vi "IQ_ramp_test.vi"() -> ()   [LabVIEW 2013]
panel:
  in  "Q ramp length":i32
  in  "I ramp length":i32
  out "signal":i16[](graph)
  out "IQ counters":dbl[][](graph)
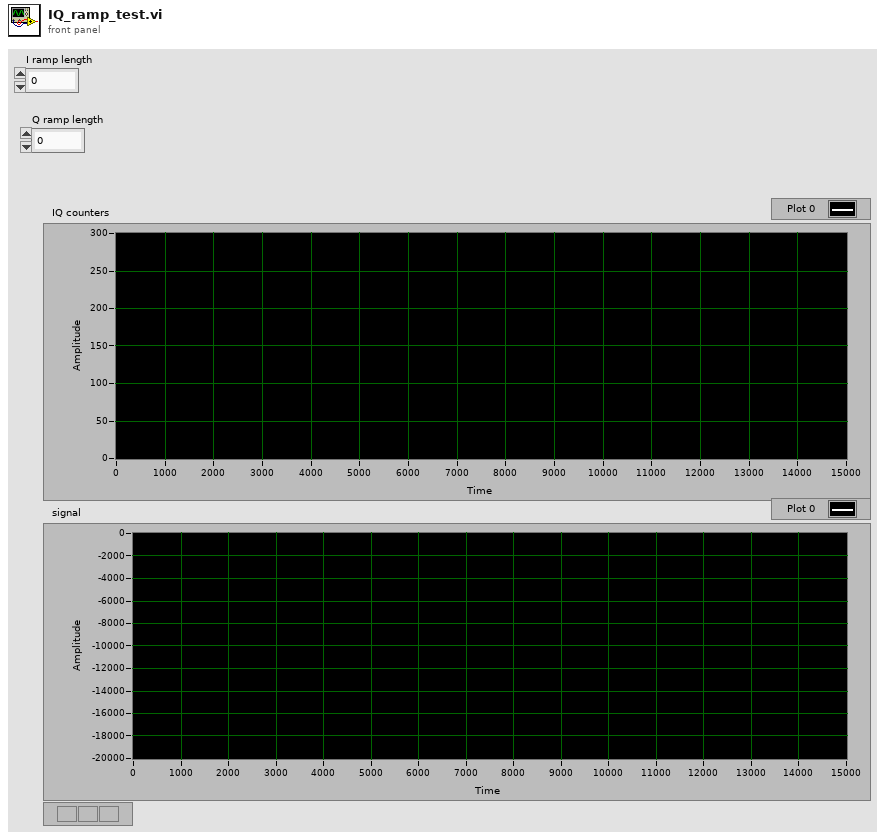
[diagram p1: front panel]
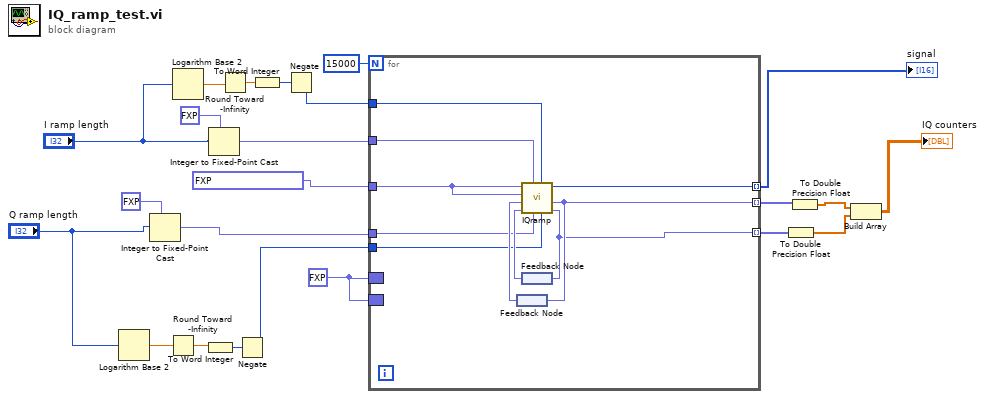
[diagram p0: block diagram]
diagram:
  w22 = fxp<+/-,32,32> 0.0 ("Q counter out")
  n1 = Logarithm Base 2(1:"Q ramp length") -> (0:w14:dbl)
  n2 = Integer to Fixed-Point Cast(fixed-point type=fxp<+/-,32,32> 0.0 ("I ramp length"), integer="Q ramp length") -> (fixed-point=w3:fxp<+/-,32,32>)
  n3 = Round Toward -Infinity(1:w14) -> (0:w13:dbl)
  n4 = Logarithm Base 2(1:"I ramp length") -> (0:w11:dbl)
  n5 = To Word Integer(number=w13) -> (16bit integer=w12:i16)
  n6 = Integer to Fixed-Point Cast(fixed-point type=fxp<+/-,32,32> 0.0 ("I ramp length"), integer="I ramp length") -> (fixed-point=w7:fxp<+/-,32,32>)
  n7 = Round Toward -Infinity(1:w11) -> (0:w10:dbl)
  n8 = Negate(x=w12) -> (-x=w1:i16)
  n9 = To Word Integer(number=w10) -> (16bit integer=w9:i16)
  n10 = Negate(x=w9) -> (-x=w2:i16)
  n11 = for {
    N: 15000 -> [_]
    tunnel: fxp<+/-,16,0> 0.4999847412109375 ("sin") -> [w33]
    border: w22 -> [_]
    border: w22 -> [_]
    tunnel: [w30] -> w21 mode=indexing
    tunnel: [w29] -> w19 mode=indexing
    tunnel: [w28] -> w18 mode=indexing
    tunnel: w2 -> [w27]
    tunnel: w3 -> [w26]
    tunnel: w1 -> [w25]
    tunnel: w7 -> [w24]
    n12 = feedback #1() -> (w31:fxp<+/-,32,32>)
    n13 = feedback #2() -> (w32:fxp<+/-,32,32>)
    n14 = call "IQramp.vi"("Q shift bits"=w25, "I shift bits"=w27, "Q ramp length"=w26, "I ramp length"=w24, "Q counter"=w32, "I counter"=w31, "cos"=w33, "sin"=w33) -> ("Q counter out"=w28:fxp<+/-,32,32>, "I counter out"=w30:fxp<+/-,32,32>, "signal"=w29:i16)  [unwired: 1 in]
    n15 = feedback-in #1(w30) -> ()
    n16 = feedback-in #2(w28) -> ()
  }
  "signal" <- w19
  n17 = To Double Precision Float(number=w18) -> (double precision float=w17:dbl[])
  n18 = To Double Precision Float(number=w21) -> (double precision float=w16:dbl[])
  n19 = Build Array(w16, w17) -> (→"IQ counters":dbl[][])
